vi "SLSC Read Properties_O2.vi"(8 "error in (no error)":errorcluster, 10 "SLSC Device":refnum<k21>, 11 "SLSC EDS module in":T1) -> (0 "error out":errorcluster, 3 "SLSC EDS module out":T1)   [LabVIEW 2017]
uses:
  SLSC EDS API/JSON parsing/EDSjsonStructure.ctl
  SLSC EDS API/JSON parsing/enum.ctl
  SLSC EDS API/JSON parsing/property.ctl
  SLSC EDS API/JSON parsing/command.ctl
  SLSC EDS API/JSON parsing/scale.ctl
  SLSC EDS API/JSON parsing/physicalChannel.ctl
  SLSC EDS API/JSON parsing/register.ctl
  <vilib>/SLSC/Initialize Session with Devices.vi
  <vilib>/SLSC/Get Generic Property (Bool).vi
  <vilib>/SLSC/Get Generic Property (String).vi
  <vilib>/SLSC/Get Generic Property (DBL).vi
  <vilib>/SLSC/Get Generic Property (I32).vi
  <vilib>/SLSC/Get Generic Property (I64).vi
  <vilib>/SLSC/Get Generic Property (U32).vi
  <vilib>/SLSC/Get Generic Property (U64).vi
  <vilib>/SLSC/Close Session.vi
  <vilib>/SLSC/SLSC.lvlib
  SLSC CD API/SLSC CD System Explorer/SLSC CD System Explorer.lvlib
  SLSC CD API/SLSC CD Shared/SLSC CD Shared.lvlib
panel:
  # "not working\nregisterMap->registers->initialValue"
  # "not working\nregisterMap->registers->initialValue"
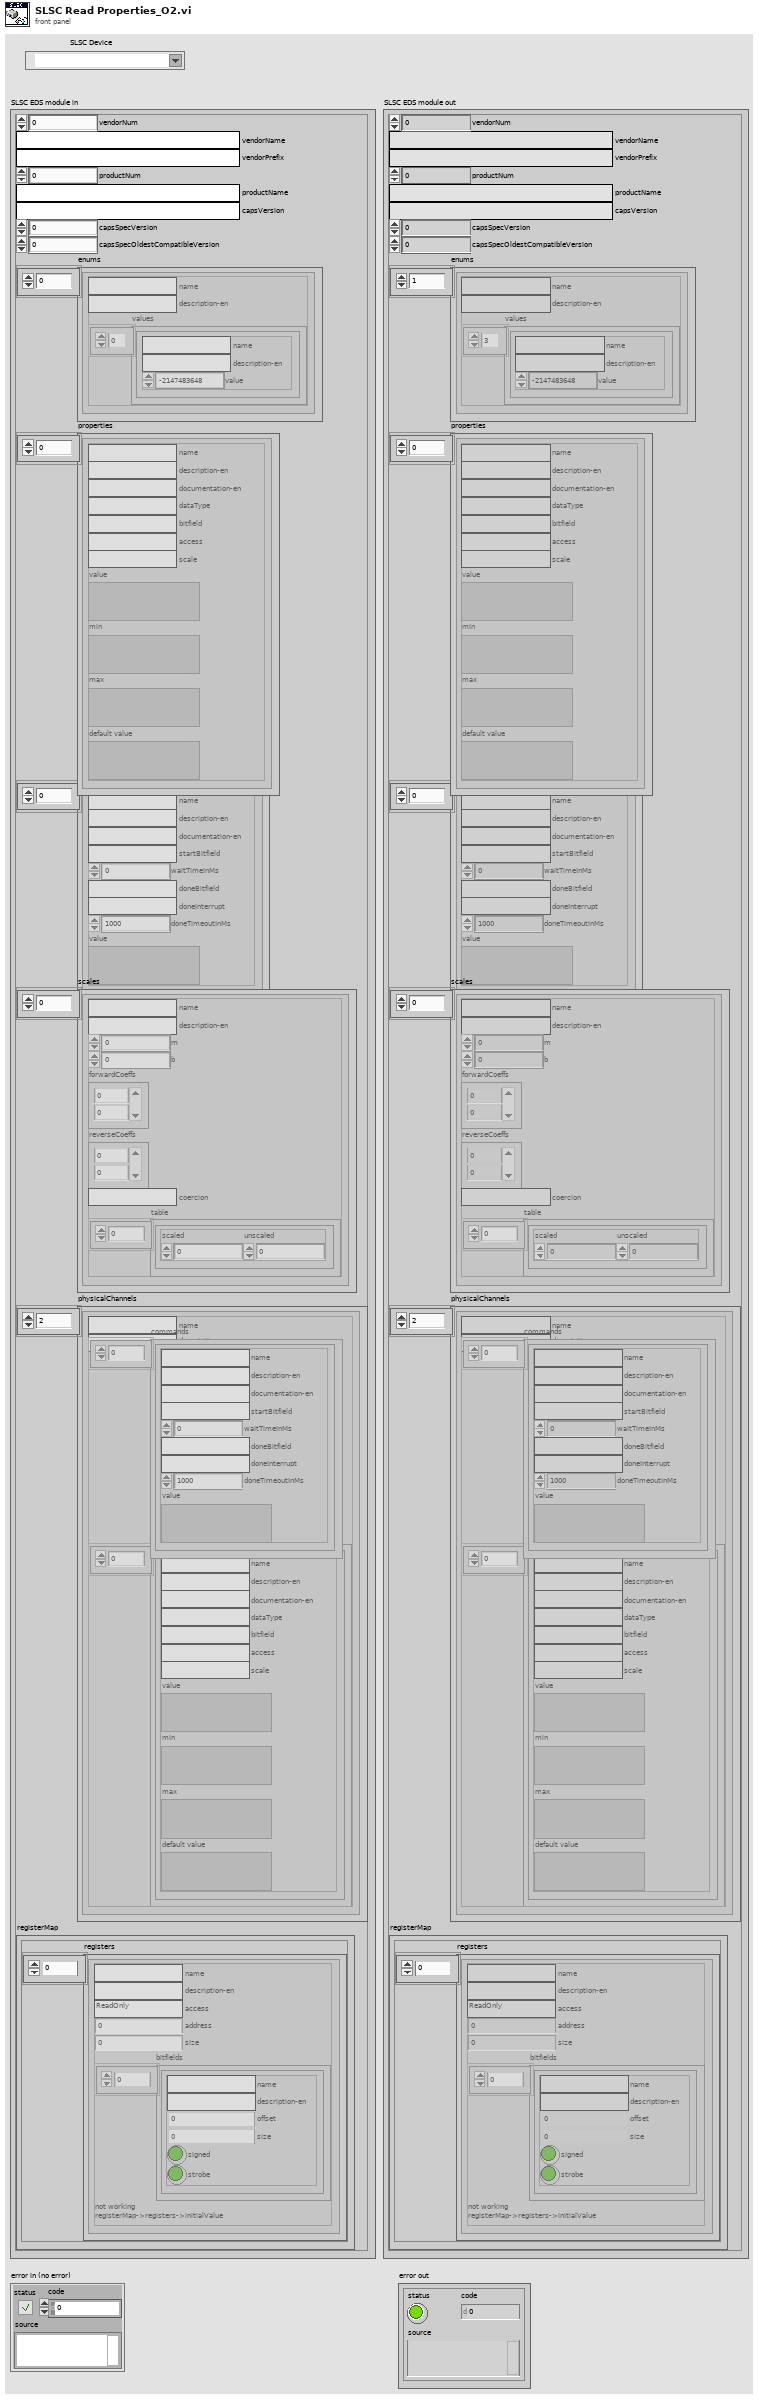
[diagram p1: front panel]
types:
  T1 = typedef "EDSjsonStructure.ctl" = cluster{"vendorNum":u32, "vendorName":string, "vendorPrefix":string, "productNum":u32, "productName":string, "capsVersion":string, "capsSpecVersion":u32, "capsSpecOldestCompatibleVersion":u32, "enums":T2[], "properties":T3[], "commands":T4[], "scales":T5[], "physicalChannels":T6[], "registerMap":cluster{"registers":T7[]}}
  T2 = typedef "enum.ctl" = cluster{"name":string, "description-en":string, "values":cluster{"name":string, "description-en":string, "value":i32}[]}
  T3 = typedef "property.ctl" = cluster{"name":string, "description-en":string, "documentation-en":string, "dataType":string, "bitfield":string, "access":string, "scale":string, "value":variant, "min":variant, "max":variant, "default value":variant}
  T4 = typedef "command.ctl" = cluster{"name":string, "description-en":string, "documentation-en":string, "startBitfield":string, "waitTimeInMs":i32, "doneBitfield":string, "doneInterrupt":string, "doneTimeoutInMs":i32, "value":variant}
  T5 = typedef "scale.ctl" = cluster{"name":string, "description-en":string, "m":dbl, "b":dbl, "forwardCoeffs":dbl[], "reverseCoeffs":dbl[], "coercion":string, "table":cluster{"scaled":dbl, "unscaled":dbl}[]}
  T6 = typedef "physicalChannel.ctl" = cluster{"name":string, "description-en":string, "commands":T4[], "properties":T3[]}
  T7 = typedef "register.ctl" = cluster{"name":string, "description-en":string, "access":string, "address":u32, "size":u32, "bitfields":cluster{"name":string, "description-en":string, "offset":u32, "size":u32, "signed":bool, "strobe":bool}[]}
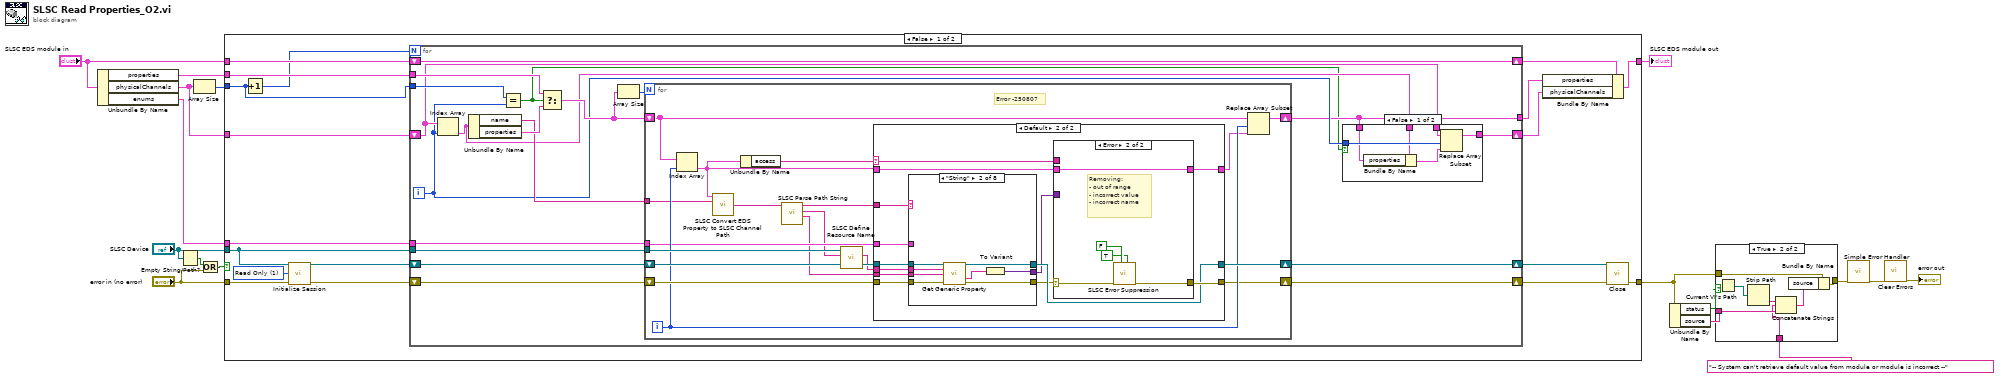
[diagram p0: block diagram]
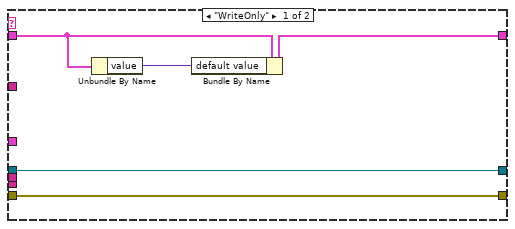
[diagram p4: hidden frame]
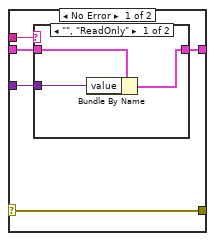
[diagram p5: hidden frame]
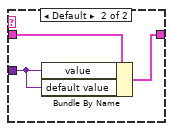
[diagram p6: hidden frame]
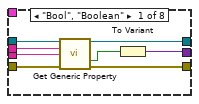
[diagram p7: hidden frame]
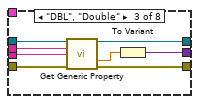
[diagram p8: hidden frame]
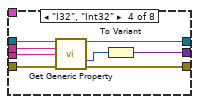
[diagram p9: hidden frame]
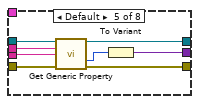
[diagram p10: hidden frame]
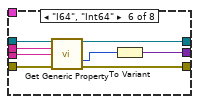
[diagram p11: hidden frame]
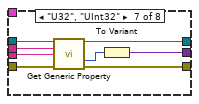
[diagram p12: hidden frame]
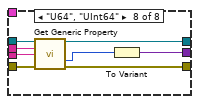
[diagram p13: hidden frame]
diagram:
  n1 = Unbundle By Name("SLSC EDS module in") -> ("properties"=w1:T3[], "physicalChannels"=w2:T6[], "enums"=w4:T2[])
  n2 = Empty String/Path?(string/path="SLSC Device") -> (empty?=w6:bool)
  n3 = Array Size(array=w2) -> (size(s)=w3:i32)
  n4 = Or(x=w6, y="error in (no error)") -> (x .or. y?=w9:bool)
  n5 = case shown="False" w9 {
    tunnel: "SLSC EDS module in" -> [w35 w179]
    tunnel: [w21 w179] -> w17
    tunnel: "SLSC Device" -> [w30 _]
    tunnel: [w32 w178] -> w14
    tunnel: "error in (no error)" -> [w28 w178]
    tunnel: w4 -> [w27 _]
    tunnel: w3 -> [w23 _]
    tunnel: w2 -> [w26 _]
    tunnel: w1 -> [w25 _]
    frame False {
      w18 = 1 items=["None"=0, "Read Only"=1, "Read/Write"=3] ("reservation access (Read/Write)")
      n6 = Increment(x=w23) -> (x+1=w24:i32)
      n7 = call-poly <vilib>:"Initialize Session.vi"("devices"=w30, "reservation access (Read/Write)"=w18, "error in (no error)"=w28) -> ("session out"=w31:refnum<k21>, "error out"=w29:errorcluster)  [unwired: 11 in]
      n8 = for {
        N: w24 -> [_]
        tunnel: w30 -> [w50]
        shift-right: [w43] -> w22
        shift-left: w35 -> [w43]
        shift-right: [w54] -> w34
        shift-left: w31 -> [w51]
        shift-right: [w53] -> w33
        shift-left: w29 -> [w49]
        tunnel: w27 -> [w48]
        tunnel: w25 -> [w47]
        tunnel: [w38] -> w20
        tunnel: w23 -> [w42]
        shift-right: [w37] -> w19
        shift-left: w26 -> [w41]
        i -> [w40]
        n9 = Index Array(array=w41, index=w40) -> (element=w39:T6)
        n10 = Unbundle By Name(w39) -> ("name"=w44:string, "properties"=w45:T3[])
        n11 = Equal?(x=w42, y=w40) -> (x = y?=w36:bool)
        n12 = Select(t=w47, s=w36, f=w45) -> (s? t:f=w46:T3[])
        n13 = Array Size(array=w46) -> (size(s)=w52:i32)
        n14 = for {
          N: w52 -> [_]
          shift-right: [w78] -> w38
          shift-left: w46 -> [w79]
          shift-right: [w76] -> w54
          shift-left: w51 -> [w73]
          tunnel: w50 -> [w71]
          tunnel: w44 -> [w64]
          tunnel: w48 -> [w65]
          shift-right: [w66] -> w53
          shift-left: w49 -> [w75]
          i -> [w70]
          # "Error -250807"
          n15 = Index Array(array=w79, index=w70) -> (element=w68:T3)
          n16 = call "SLSC Convert EDS Property to SLSC Channel Path.vi"("property"=w68, "Physical Channel"=w64) -> ("SLSC Channel Path"=w74:string)  [unwired: 8 in, 5 out]
          n17 = Unbundle By Name(w68) -> ("access"=w69:string)
          n18 = call "SLSC Parse Path String.vi"("SLSC Channel Path"=w74) -> ("Property or Command"=w62:string, "Physical Channel"=w63:string, "Datatype"=w77:string)  [unwired: 7 in, 1 out]
          n19 = call "SLSC Define Resource Name.vi"("SLSC Item"=w63, "SLSC Module Name"=w71) -> ("Resource"=w72:string)  [unwired: 9 in]
          n20 = case shown="Default" w69 {
            selector: w69 -> [_ w87]
            tunnel: w77 -> [_ w88]
            tunnel: [w84 w89] -> w76
            tunnel: w75 -> [w83 w97]
            tunnel: [w83 w90] -> w66
            tunnel: w62 -> [_ w96]
            tunnel: w73 -> [w84 w95]
            tunnel: w72 -> [_ w94]
            tunnel: w68 -> [w81 w93]
            tunnel: [w82 w92] -> w67
            tunnel: w65 -> [_ w91]
            frame "WriteOnly" {
              n21 = Unbundle By Name(w81) -> ("value"=w80:variant)
              n22 = Bundle By Name(cluster=w81, "default value"=w80) -> (w82:T3)
            }
            frame Default {
              n23 = case shown="\"String\"" w88 {
                tunnel: w95 -> [w121 w129 w137 w145 w153 w161 w169 w177]
                tunnel: [w120 w128 w136 w144 w152 w160 w168 w176] -> w89
                tunnel: w96 -> [w119 w127 w135 w143 w151 w159 w167 w175]
                tunnel: w97 -> [w118 w126 w134 w142 w150 w158 w166 w174]
                tunnel: [w117 w125 w133 w141 w149 w157 w165 w173] -> w85
                tunnel: [w114 w122 w130 w140 w148 w156 w164 w170] -> w86
                tunnel: w94 -> [w116 w124 w131 w138 w146 w154 w162 w172]
                tunnel: w91 -> [_ _ _ _ _ _ _ _]
                frame "Bool", "Boolean" {
                  n24 = call-poly <vilib>:"Get Generic Property.vi"("session in"=w121, "resources"=w116, "property"=w119, "error in (no error)"=w118) -> ("session out"=w120:refnum<k21>, "property value"=w115:bool, "error out"=w117:errorcluster)  [unwired: 9 in]
                  n25 = To Variant(anything=w115) -> (Variant=w114:variant)
                }
                frame "String" {
                  n26 = call-poly <vilib>:"Get Generic Property.vi"("session in"=w129, "resources"=w124, "property"=w127, "error in (no error)"=w126) -> ("session out"=w128:refnum<k21>, "property value"=w123:string, "error out"=w125:errorcluster)  [unwired: 9 in]
                  n27 = To Variant(anything=w123) -> (Variant=w122:variant)
                }
                frame "DBL", "Double" {
                  n28 = call-poly <vilib>:"Get Generic Property.vi"("session in"=w137, "resources"=w131, "property"=w135, "error in (no error)"=w134) -> ("session out"=w136:refnum<k21>, "property value"=w132:dbl, "error out"=w133:errorcluster)  [unwired: 9 in]
                  n29 = To Variant(anything=w132) -> (Variant=w130:variant)
                }
                frame "I32", "Int32" {
                  n30 = call-poly <vilib>:"Get Generic Property.vi"("session in"=w145, "resources"=w138, "property"=w143, "error in (no error)"=w142) -> ("session out"=w144:refnum<k21>, "property value"=w139:i32, "error out"=w141:errorcluster)  [unwired: 9 in]
                  n31 = To Variant(anything=w139) -> (Variant=w140:variant)
                }
                frame Default {
                  n32 = call-poly <vilib>:"Get Generic Property.vi"("session in"=w153, "resources"=w146, "property"=w151, "error in (no error)"=w150) -> ("session out"=w152:refnum<k21>, "property value"=w147:i32, "error out"=w149:errorcluster)  [unwired: 9 in]
                  n33 = To Variant(anything=w147) -> (Variant=w148:variant)
                }
                frame "I64", "Int64" {
                  n34 = call-poly <vilib>:"Get Generic Property.vi"("session in"=w161, "resources"=w154, "property"=w159, "error in (no error)"=w158) -> ("session out"=w160:refnum<k21>, "property value"=w155:i64, "error out"=w157:errorcluster)  [unwired: 9 in]
                  n35 = To Variant(anything=w155) -> (Variant=w156:variant)
                }
                frame "U32", "UInt32" {
                  n36 = call-poly <vilib>:"Get Generic Property.vi"("session in"=w169, "resources"=w162, "property"=w167, "error in (no error)"=w166) -> ("session out"=w168:refnum<k21>, "property value"=w163:u32, "error out"=w165:errorcluster)  [unwired: 9 in]
                  n37 = To Variant(anything=w163) -> (Variant=w164:variant)
                }
                frame "U64", "UInt64" {
                  n38 = call-poly <vilib>:"Get Generic Property.vi"("session in"=w177, "resources"=w172, "property"=w175, "error in (no error)"=w174) -> ("session out"=w176:refnum<k21>, "property value"=w171:u64, "error out"=w173:errorcluster)  [unwired: 9 in]
                  n39 = To Variant(anything=w171) -> (Variant=w170:variant)
                }
              }
              n40 = case shown="Error" w85 {
                selector: w85 -> [w100 w112]
                tunnel: w93 -> [w102 w113]
                tunnel: [w101 w113] -> w92
                tunnel: w86 -> [w99 _]
                tunnel: [w100 w111] -> w90
                tunnel: w87 -> [w98 _]
                frame No Error {
                  n41 = case shown="\"\", \"ReadOnly\"" w98 {
                    tunnel: w102 -> [w105 w108]
                    tunnel: [w104 w107] -> w101
                    tunnel: w99 -> [w103 w106]
                    frame "", "ReadOnly" {
                      n42 = Bundle By Name(cluster=w105, "value"=w103) -> (w104:T3)
                    }
                    frame Default {
                      n43 = Bundle By Name(cluster=w108, "value"=w106, "default value"=w106) -> (w107:T3)
                    }
                  }
                }
                frame Error {
                  # "Removing: \n- out of range\n- incorrect value\n- incorrect name"
                  n44 = call "SLSC Error Suppression.vi"("error in (no error)"=w112, "Popup Error?"=FALSE, "Clear All Error?"=TRUE) -> ("error out"=w111:errorcluster)  [unwired: 6 in, 1 out]
                }
              }
            }
          }
          n45 = Replace Array Subset(array=w79, new element=w67, index=w70) -> (w78:T3[])
        }
        n46 = case shown="False" w36 {
          tunnel: w41 -> [w60 w61]
          tunnel: w40 -> [w59 _]
          tunnel: w39 -> [w58 _]
          tunnel: w38 -> [w57 _]
          tunnel: [w55 w61] -> w37
          frame False {
            n47 = Bundle By Name(cluster=w58, "properties"=w57) -> (w56:T6)
            n48 = Replace Array Subset(array=w60, new element=w56, index=w59) -> (w55:T6[])
          }
          frame True {
          }
        }
      }
      n49 = Bundle By Name(cluster=w22, "properties"=w20, "physicalChannels"=w19) -> (w21:T1)
      n50 = call-poly <vilib>:"Close.vi"("session in"=w34, "error in (no error)"=w33) -> ("error out"=w32:errorcluster)  [unwired: 13 in]
    }
    frame True {
    }
  }
  "SLSC EDS module out" <- w17
  n51 = Unbundle By Name(w14) -> ("status"=w11:bool, "source"=w12:string)
  n52 = case shown="True" w11 {
    tunnel: w14 -> [w180 w187]
    tunnel: [w180 w186] -> w13
    tunnel: w12 -> [_ w185]
    tunnel: "-- System can't retrieve default value from module or module is incorrect --" -> [_ w183]
    frame False {
    }
    frame True {
      n53 = Current VI's Path() -> (path=w182:path)
      n54 = Strip Path(path=w182) -> (name=w181:string)  [unwired: 1 out]
      n55 = Concatenate Strings(w181, w183, w185) -> (w184:string)
      n56 = Bundle By Name(cluster=w187, "source"=w184) -> (w186:errorcluster)
    }
  }
  n57 = call <vilib>:"Simple Error Handler.vi"("error in (no error)"=w13) -> ("error out"=w16:errorcluster)  [unwired: 4 in, 4 out]
  n58 = call <vilib>:"Clear Errors.vi"("error in (no error)"=w16) -> ("error out"=→"error out":errorcluster)  [unwired: 5 in, 1 out]
